vi "TCP-IMG-Receiver.vi"() -> ()   [LabVIEW 2019]
panel:
  out "Image":T1(plugin-control)
  in  "Stop":bool
  # "TCP Image Receiver"
  # "Instructions:\n1.  Run \"TCP-IMG-Sender\".\n2. Run this VI.\n3. See the images received via TCP."
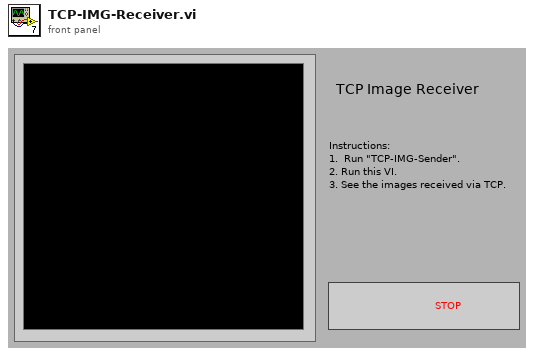
[diagram p1: front panel]
types:
  T1 = typedef "IMAQ Image.ctl" = refnum<image>
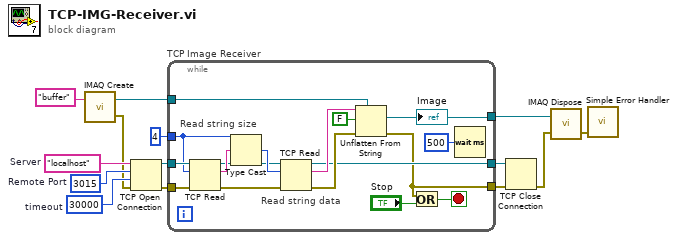
[diagram p0: block diagram]
diagram:
  w2 = 30000  # timeout
  w3 = "localhost"  # Server
  w14 = u16 3015  # Remote Port
  n1 = call "IMAQ Create"("Image Name"="buffer") -> ("New Image"=w12:T1, "error out"=w1:errorcluster)  [unwired: 4 in]
  n2 = TCP Open Connection(address=w3, remote port or service name=w14, timeout ms (60000)=w2, error in (no error)=w1) -> (connection ID=w5:refnum<k5>, error out=w4:errorcluster)  [unwired: 1 in]
  n3 = while "TCP Image Receiver" {
    tunnel: w5 -> [w27]
    tunnel: w12 -> [w24]
    tunnel: [w16] -> w11
    tunnel: 4 -> [w22]
    tunnel: [w21] -> w8
    tunnel: w4 -> [w18]
    tunnel: [w17] -> w6
    stop <- w19 stop-if-true
    # "Read string data"
    # "Read string size"
    n4 = TCP Read(connection ID=w27, bytes to read=w22, error in (no error)=w18) -> (connection ID out=w29:refnum<k5>, data out=w31:string, error out=w28:errorcluster)  [unwired: 2 in]
    n5 = Type Cast(type=w22, x=w31) -> (*(type *) &x=w30:i32)
    n6 = TCP Read(connection ID=w29, bytes to read=w30, error in (no error)=w28) -> (connection ID out=w21:refnum<k5>, data out=w26:string, error out=w23:errorcluster)  [unwired: 2 in]
    n7 = Unflatten From String(type=w24, binary string=w26, data includes array or string size? (T)=FALSE, error in (no error)=w23) -> (value=w16:T1, error out=w17:errorcluster)  [unwired: 1 in, 1 out]
    "Image" <- w16
    n8 = Or(x=w17, y="Stop") -> (x .or. y?=w19:bool)
    n9 = Wait (ms)(milliseconds to wait=u32 500) -> ()  [unwired: 1 out]
  }
  n10 = TCP Close Connection(connection ID=w8, error in (no error)=w6) -> (error out=w9:errorcluster)  [unwired: 1 in, 1 out]
  n11 = call "IMAQ Dispose"("Image"=w11, "error in (no error)"=w9) -> ("error out"=w7:errorcluster)  [unwired: 4 in]
  n12 = call <vilib>:"Simple Error Handler.vi"("error in (no error)"=w7) -> ()  [unwired: 4 in, 5 out]
